vi "Actor Core.vi"(8 "error in":errorcluster, 11 "Caller in":refnum<class "Actor.lvclass">) -> (0 "error out":errorcluster, 3 "Actor out":refnum<class "Actor.lvclass">)   [LabVIEW 2020, in "Actor.lvlib" / "Actor.lvclass"]
doc: "(<B>Filename</B>: Actor Framework.lvlib:Actor.lvclass:Actor Core.vi)\n\nReceives messages to the actor, reacts to them, and initiates any error handling that may shut the actor down.\n\nDescendant classes may override this VI to append parallel tasks for the actor to complete while it handles messages. Overrides use the Call Parent Class Method node."
uses:
  Actor.lvclass
  <vilib>/ActorFramework/Actor/Actor.lvclass
  Actor.lvclass/Actor.ctl
  <vilib>/ActorFramework/Message Enqueuer/Message Enqueuer.lvclass/Message Enqueuer.ctl
  <vilib>/ActorFramework/Message Enqueuer/Enqueue.vi
  <vilib>/ActorFramework/Stop Msg/Stop Msg.lvclass
  C:/Program Files/National Instruments/LabVIEW 2020/vi.lib/ActorFramework/Message/Message.lvclass
  <vilib>/ActorFramework/Message Priority Queue/Priority Enqueue.vi
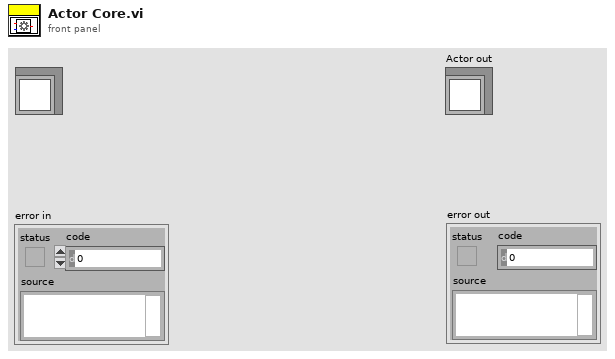
[diagram p1: front panel]
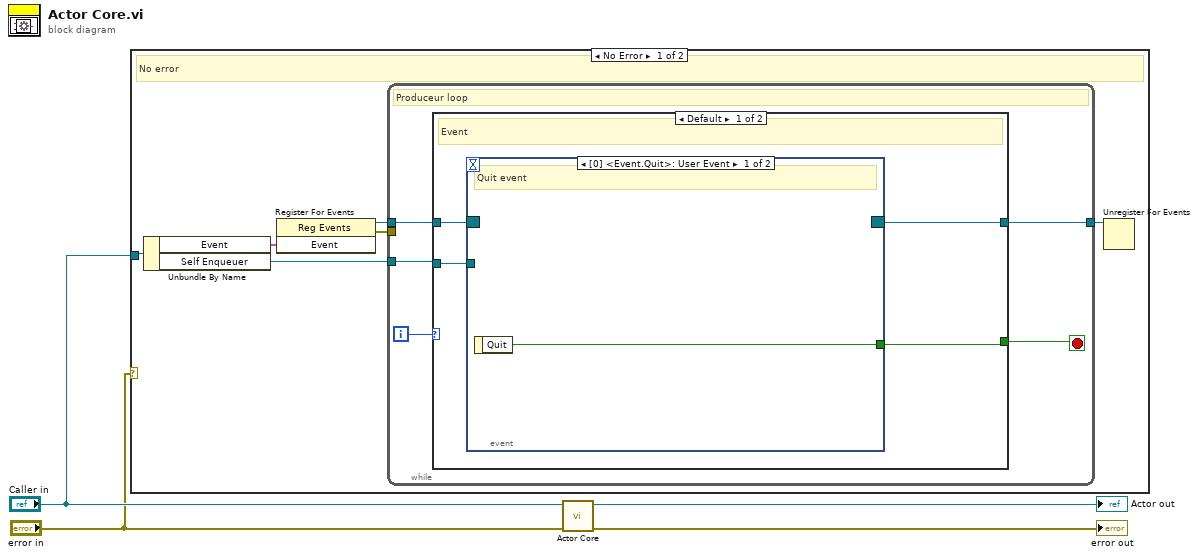
[diagram p0: block diagram]
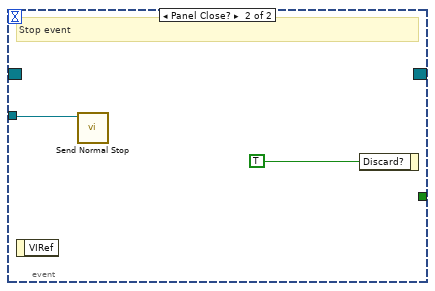
[diagram p2: hidden frame]
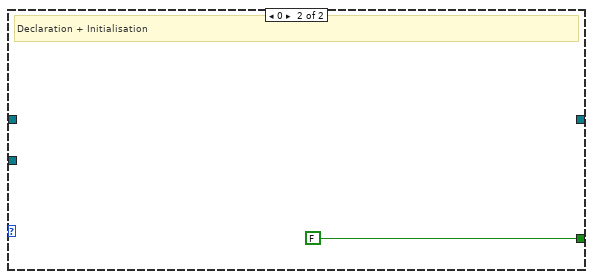
[diagram p3: hidden frame]
diagram:
  n1 = case shown="No Error" "error in" {
    tunnel: "Caller in" -> [w8 _]
    frame No Error {
      # "No error"
      n2 = Unbundle By Name(w8) -> ("Event"=w6:cluster{"Quit":refnum<user-event>}, "Self Enqueuer"=w9:refnum<class "Message Enqueuer.lvclass">)
      n3 = register-events(w6) -> (reference out=w7:refnum<event-registration>, error out=w5:errorcluster)  [unwired: 2 in]
      n4 = while {
        tunnel: [w13] -> w10
        tunnel: w9 -> [w12]
        tunnel: w7 -> [w11]
        tunnel: w5 -> [_]
        i -> [w15]
        stop <- w14 stop-if-true
        # "Produceur loop"
        n5 = case shown="Default" w15 {
          tunnel: w12 -> [w17 _]
          tunnel: [w18 FALSE] -> w14
          tunnel: [w19 _] -> w13
          tunnel: w11 -> [w16 _]
          frame Default {
            # "Event"
            n6 = event shown="[0] <Event.Quit>: User Event" {
              selector: w16 -> [_ _]
              dyn-events: [_ _] -> w19
              timeout: _ -> [_ _]
              tunnel: [w20 _] -> w18
              tunnel: w17 -> [_ w21]
              event User Event {
                # "Quit event"
                n7 = event-data() -> ("Quit"=w20:bool)  [unwired: 1 in]
              }
              event Panel Close? {
                # "Stop event"
                n8 = event-data() -> ()  [unwired: 1 in, 1 out]
                n9 = call <vilib>:"Send Normal Stop.vi"("Message Enqueuer"=w21) -> ()  [unwired: 10 in, 1 out]
                n10 = event-data("Discard?"=TRUE) -> ()  [unwired: 1 in, 1 out]
              }
            }
          }
          frame 0 {
            # "Declaration + Initialisation"
          }
        }
      }
      n11 = Unregister For Events(event registration refnum=w10) -> ()  [unwired: 1 in, 1 out]
    }
    frame Error {
    }
  }
  n12 = call-parent "Actor Core.vi"("error in"="error in", "Actor in"="Caller in") -> ("error out"=→"error out":errorcluster, "Actor out"=→"Actor out":refnum<class "Actor.lvclass">)  [unwired: 8 in]
